vi "b.vi"   [LabVIEW 2020]
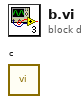
[diagram p0: block diagram]
diagram:
  n1 = call "c.vi"() -> ()  [unwired: 12 in]
